vi "Append Sweep Waveforms.vi"(8 "error in (no error)":errorcluster, 10 "New SweepWaveforms":T1, 11 "SweepWaveforms in":T1) -> (0 "error out":errorcluster, 3 "SweepWaveforms out":T1)   [LabVIEW 2019, in "Instrument.Lockin.lvlib" / "Instrument.DAQ.lvclass"]
uses:
  Instrument.DAQ.lvclass
  Typedefs/PublicEvents--DAQ.getSweepWaveforms.ctl
  Waveform.Attributes/Waveform.Attributes.lvlib
  Generator/Generator.lvclass
panel:
  out "Waveform Graph":waveform(dbl)[](graph)
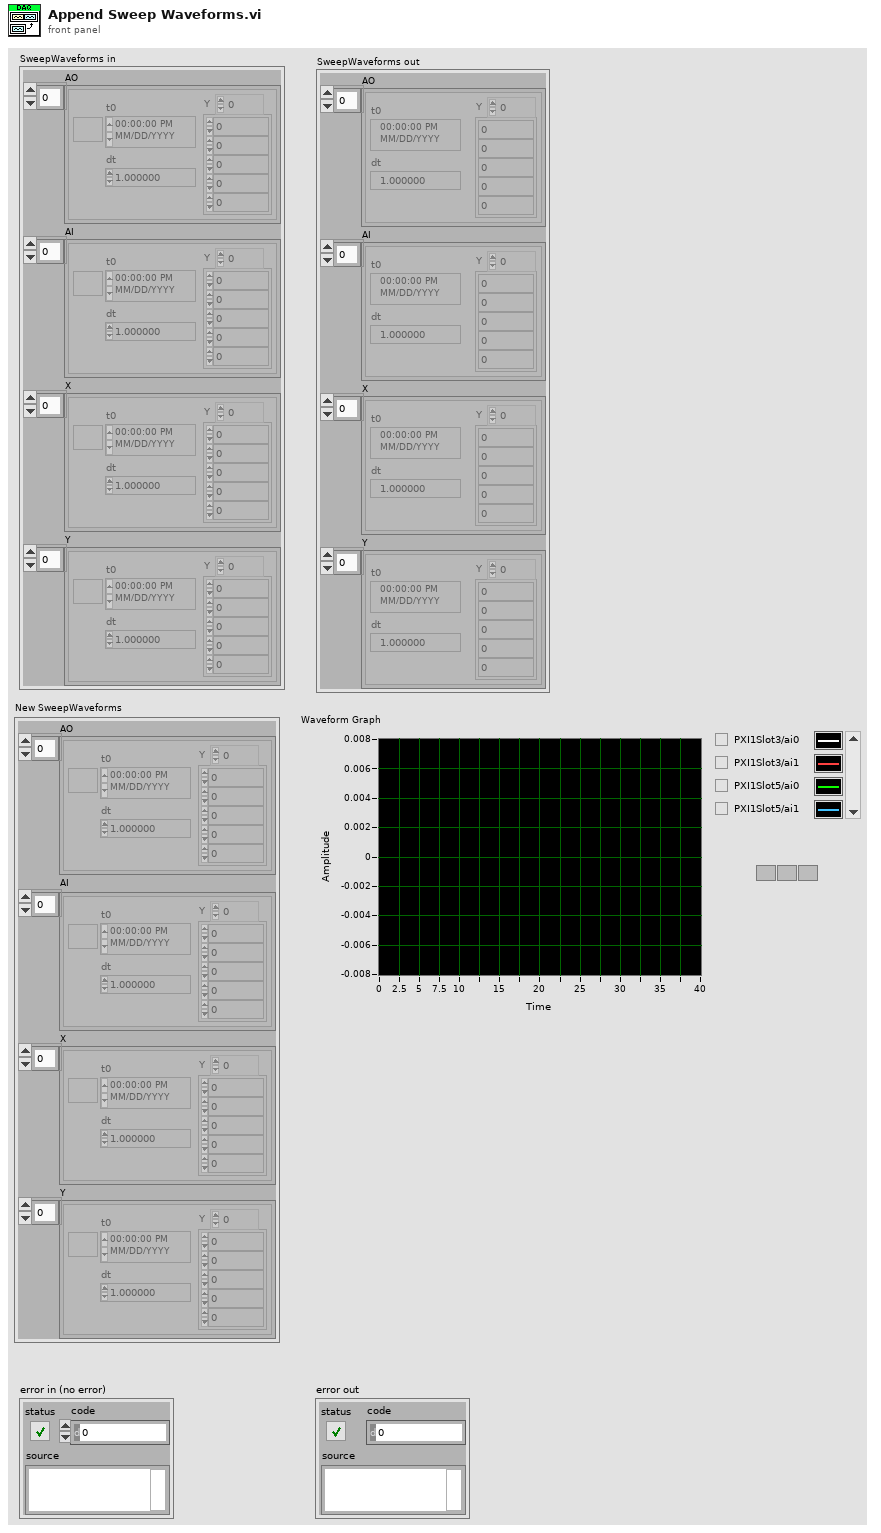
[diagram p1: front panel]
types:
  T1 = typedef "Instrument.Lockin.lvlib/Instrument.DAQ.lvclass/PublicEvents--DAQ.getSweepWaveforms.ctl" = cluster{"AO":waveform(dbl)[], "AI":waveform(dbl)[], "X":waveform(dbl)[], "Y":waveform(dbl)[]}
  T2 = typedef "Generator.lvclass/Generator.Sweep Status--enum.ctl" = enum16{"idle", "initializing", "waiting", "sweeping", "stopping"}
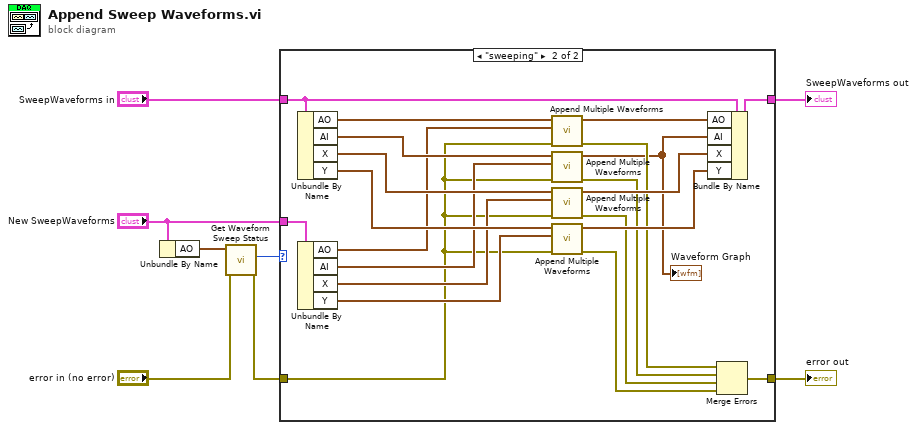
[diagram p0: block diagram]
diagram:
  n1 = Unbundle By Name("New SweepWaveforms") -> ("AO"=w5:waveform(dbl)[])
  n2 = call "Get Waveform Sweep Status.vi"("error in (no error)"="error in (no error)", "Waveforms in"=w5) -> ("error out"=w3:errorcluster, "sweep status"=w2:T2)  [unwired: 7 in, 1 out]
  n3 = case shown="\"sweeping\"" w2 {
    tunnel: [w9 w25] -> w8
    tunnel: "SweepWaveforms in" -> [w9 w24]
    tunnel: [w10 w23] -> w6
    tunnel: w3 -> [w10 w17]
    tunnel: "New SweepWaveforms" -> [_ w21]
    frame Default {
    }
    frame "sweeping" {
      n4 = Unbundle By Name(w24) -> ("AO"=w22:waveform(dbl)[], "AI"=w27:waveform(dbl)[], "X"=w28:waveform(dbl)[], "Y"=w29:waveform(dbl)[])
      n5 = Unbundle By Name(w21) -> ("AO"=w12:waveform(dbl)[], "AI"=w20:waveform(dbl)[], "X"=w19:waveform(dbl)[], "Y"=w18:waveform(dbl)[])
      n6 = call "Append Multiple Waveforms.vi"("error in (no error)"=w17, "Waveform B []"=w12, "Waveforrm A []"=w22) -> ("error out"=w13:errorcluster, "Waveform out []"=w26:waveform(dbl)[])  [unwired: 7 in]
      n7 = call "Append Multiple Waveforms.vi"("error in (no error)"=w17, "Waveform B []"=w20, "Waveforrm A []"=w27) -> ("error out"=w14:errorcluster, "Waveform out []"=w11:waveform(dbl)[])  [unwired: 7 in]
      "Waveform Graph" <- w11
      n8 = call "Append Multiple Waveforms.vi"("error in (no error)"=w17, "Waveform B []"=w19, "Waveforrm A []"=w28) -> ("error out"=w15:errorcluster, "Waveform out []"=w30:waveform(dbl)[])  [unwired: 7 in]
      n9 = call "Append Multiple Waveforms.vi"("error in (no error)"=w17, "Waveform B []"=w18, "Waveforrm A []"=w29) -> ("error out"=w16:errorcluster, "Waveform out []"=w31:waveform(dbl)[])  [unwired: 7 in]
      n10 = Bundle By Name(cluster=w24, "AO"=w26, "AI"=w11, "X"=w30, "Y"=w31) -> (w25:T1)
      n11 = Merge Errors(w13, w14, w15, w16) -> (w23:errorcluster)
    }
  }
  "SweepWaveforms out" <- w8
  "error out" <- w6
